vi "libssh2_hostkey_hash.vi"(8 "error in (no error)":errorcluster, 10 "hash_type":i32=2, 11 "Session":T1) -> (0 "error out":errorcluster, 3 "return value":string)   [LabVIEW 2013, in "libssh2.lvlib"]
uses:
  libssh2.lvlib
  Session Refnum.ctl
  libssh2.dll
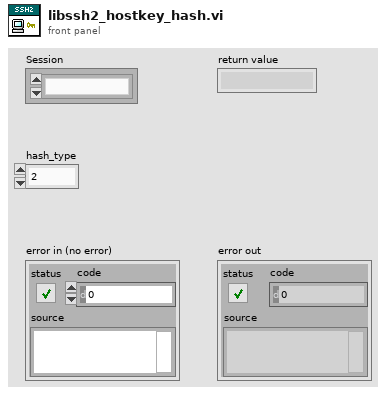
[diagram p1: front panel]
types:
  T1 = typedef "libssh2.lvlib/Session Refnum.ctl" = refnum<k1>
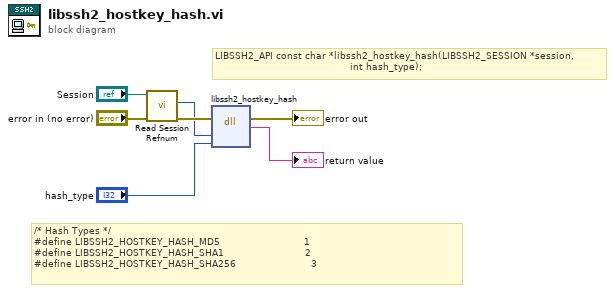
[diagram p0: block diagram]
diagram:
  # "/* Hash Types */\n#define LIBSSH2_HOSTKEY_HASH_MD5                            1\n#define LIBSSH2_HOSTKEY_HASH_SHA1                           2\n#define LIBSSH2_HOSTKEY_HASH_SHA256                         3"
  # "LIBSSH2_API const char *libssh2_hostkey_hash(LIBSSH2_SESSION *session,\n                                             int hash_type);"
  n1 = call "Read Session Refnum.vi"("error in (no error)"="error in (no error)", "Session"="Session") -> ("error out"=w3:errorcluster, "LIBSSH2_SESSION*"=w1:u64)  [unwired: 8 in]
  n2 = dll-call lib="C:/Users/pasca/source/repos/libssh2-labview/libssh2**.*" fn="libssh2_hostkey_hash"(error in=w3, "session"=w1, "hash_type"="hash_type") -> (error out=→"error out":errorcluster, "return value"=→"return value":string)  [unwired: 4 in, 1 out]
